vi "RP100.Set Level.vi"(8 "error in (no error)":errorcluster, 9 "Level (V)":dbl, 10 "Output Channel":T1, 11 "VISA resource name":refnum<visa-resource-name>) -> (0 "error out":errorcluster, 2 "Output Channel":T1, 3 "VISA Refnum out":refnum<visa-resource-name>)   [LabVIEW 2016, in "RP100.lvclass"]
uses:
  RP100.lvclass
  Typedefs/Output Channel--Enum.ctl
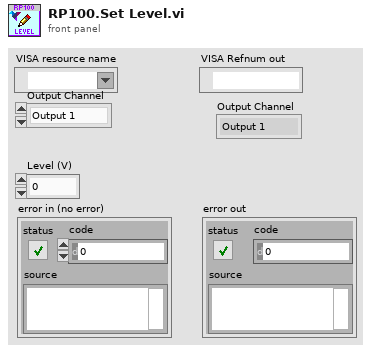
[diagram p1: front panel]
types:
  T1 = typedef "RP100.lvclass/Output Channel--Enum.ctl" = enum16{"Output 1", "Output 2"}
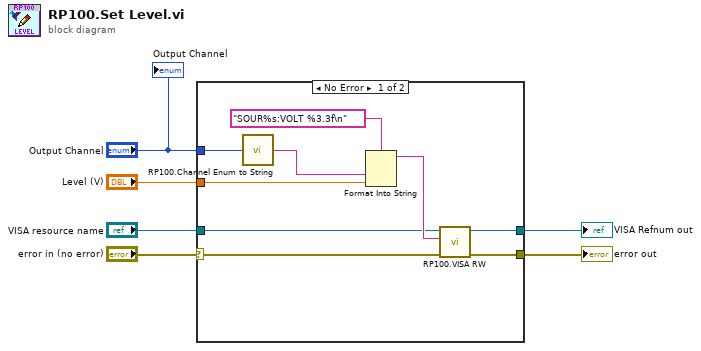
[diagram p0: block diagram]
diagram:
  n1 = case shown="No Error" "error in (no error)" {
    selector: "error in (no error)" -> [w7 w17]
    tunnel: [w15 w16] -> w6
    tunnel: "Level (V)" -> [w14 _]
    tunnel: "VISA resource name" -> [w12 w16]
    tunnel: "Output Channel" -> [w9 _]
    tunnel: [w11 w17] -> w2
    frame No Error {
      n2 = call "RP100.Channel Enum to String.vi"("OutputChannel"=w9) -> ("format string"=w8:string)
      n3 = Format Into String(format string="SOUR%s:VOLT %3.3f\n", w8, w14) -> (resulting string=w13:string)  [unwired: 2 in, 1 out]
      n4 = call "RP100.VISA RW.vi"("error in (no error)"=w7, "Write"=w13, "VISA Refnum in"=w12) -> ("error out"=w11:errorcluster, "VISA Refnum out"=w15:refnum<visa-resource-name>)  [unwired: 6 in, 1 out]
    }
    frame Error {
    }
  }
  "error out" <- w2
  "VISA Refnum out" <- w6
  "Output Channel" <- "Output Channel"
